vi "Create Session.vi"(5 "net-http-client (type)":refnum<class "net-http-client.lvclass">, 6 "verify server (true)":bool, 7 "cookie file":path, 8 "error in (no error)":errorcluster, 9 "password":string, 10 "username":string) -> (0 "error out":errorcluster, 3 "net-http-client out":refnum<class "net-http-client.lvclass">)   [LabVIEW 2020, in "net-http-client.lvclass"]
uses:
  net-http-client.lvclass
  <vilib>/Viviota/Viviota HTTP Client NET/LabVIEWHTTPClient_NET/HttpClient_NET.lvclass
  net-http-client.lvclass/net-http-client.ctl
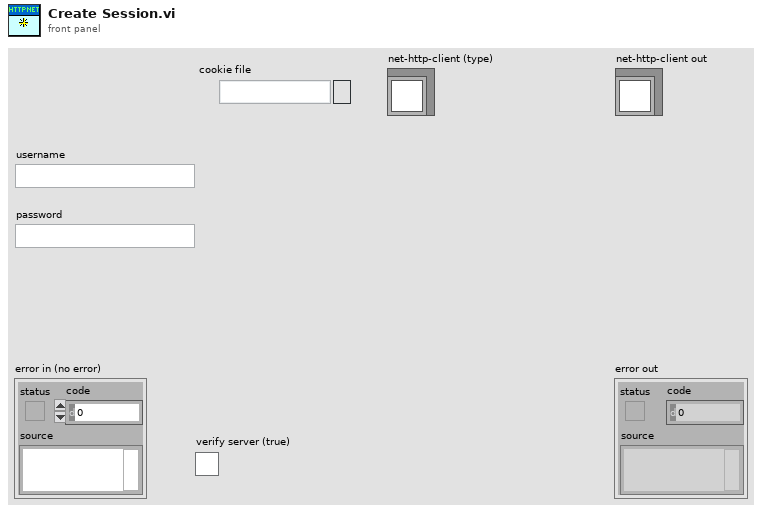
[diagram p1: front panel]
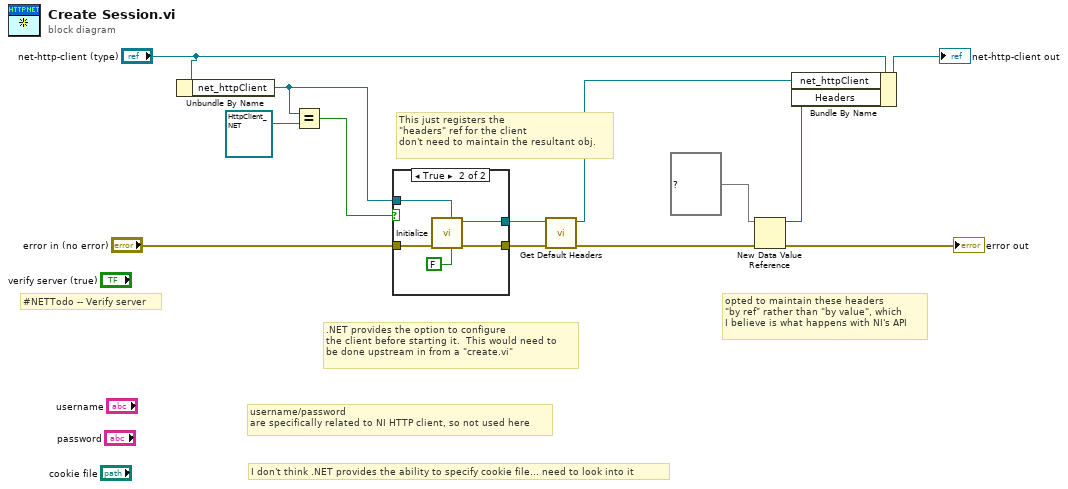
[diagram p0: block diagram]
diagram:
  # "This just registers the \n\"headers\" ref for the client\ndon't need to maintain the resultant obj."
  # "opted to maintain these headers\n\"by ref\" rather than \"by value\", which\nI believe is what happens with NI's API"
  # ".NET provides the option to configure\nthe client before starting it.  This would need to \nbe done upstream in from a \"create.vi\""
  # "I don't think .NET provides the ability to specify cookie file... need to look into it"
  # "username/password\nare specifically related to NI HTTP client, so not used here"
  # "#NETTodo -- Verify server"
  n1 = Unbundle By Name("net-http-client (type)") -> ("net_httpClient"=w5:refnum<class "HttpClient_NET.lvclass">)
  n2 = Equal?(x=w5, y=refnum<class "HttpClient_NET.lvclass"> refnum ("net_httpclient")) -> (x = y?=w6:bool)
  n3 = case shown="True" w6 {
    tunnel: "error in (no error)" -> [w14 w20]
    tunnel: [w14 w19] -> w10
    tunnel: [w15 w18] -> w9
    tunnel: w5 -> [w15 w16]
    frame False {
    }
    frame True {
      n4 = call <vilib>:"Initialize.vi"("Allow Handler Configuration [F]"=FALSE, "HTTP Client In"=w16, "error in (no error)"=w20) -> ("error out"=w19:errorcluster, "HTTP Client Out"=w18:refnum<class "HttpClient_NET.lvclass">)  [unwired: 7 in]
    }
  }
  n5 = call <vilib>:"Get Default Headers.vi"("error in (no error)"=w10, "LabVIEWHTTPClient_NET in"=w9) -> ("error out"=w2:errorcluster, "LabVIEWHTTPClient_NET out"=w8:refnum<class "HttpClient_NET.lvclass">)  [unwired: 7 in, 1 out]
  n6 = New Data Value Reference(data value=map{string, string} {} ("map"), error in=w2) -> (data value reference=w4:refnum<data-value>, error out=→"error out":errorcluster)
  n7 = Bundle By Name(cluster="net-http-client (type)", "net_httpClient"=w8, "Headers"=w4) -> (→"net-http-client out":refnum<class "net-http-client.lvclass">)
